vi "ArrayToHexString.vi"(11 "U32 Array":u32[](array[numeric]) format="%.0x") -> (3 "String":string)   [LabVIEW 2017]
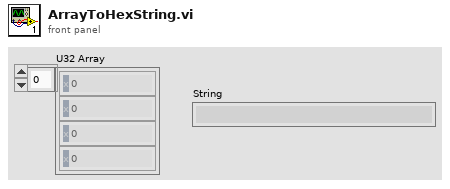
[diagram p1: front panel]
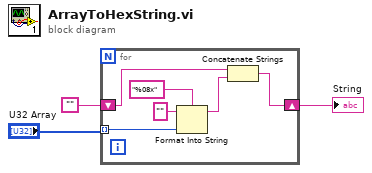
[diagram p0: block diagram]
diagram:
  n1 = for {
    tunnel: "U32 Array" -> [w7] mode=indexing
    shift-right: [w4] -> w3
    shift-left: "" -> [w6]
    n2 = Format Into String(format string="%08x", initial string="", w7) -> (resulting string=w5:string)  [unwired: 1 in, 1 out]
    n3 = Concatenate Strings(w6, w5) -> (w4:string)
  }
  "String" <- w3
